vi "FTW-CodeGen-GetTerminals.vi"(0 "PrototypeVI":refnum<vi>, 11 "error in":errorcluster) -> (4 "Terms":T1(array[cluster]), 15 "error out":errorcluster)   [LabVIEW 2014]
panel:
  # "Inputs"
  # "Outputs"
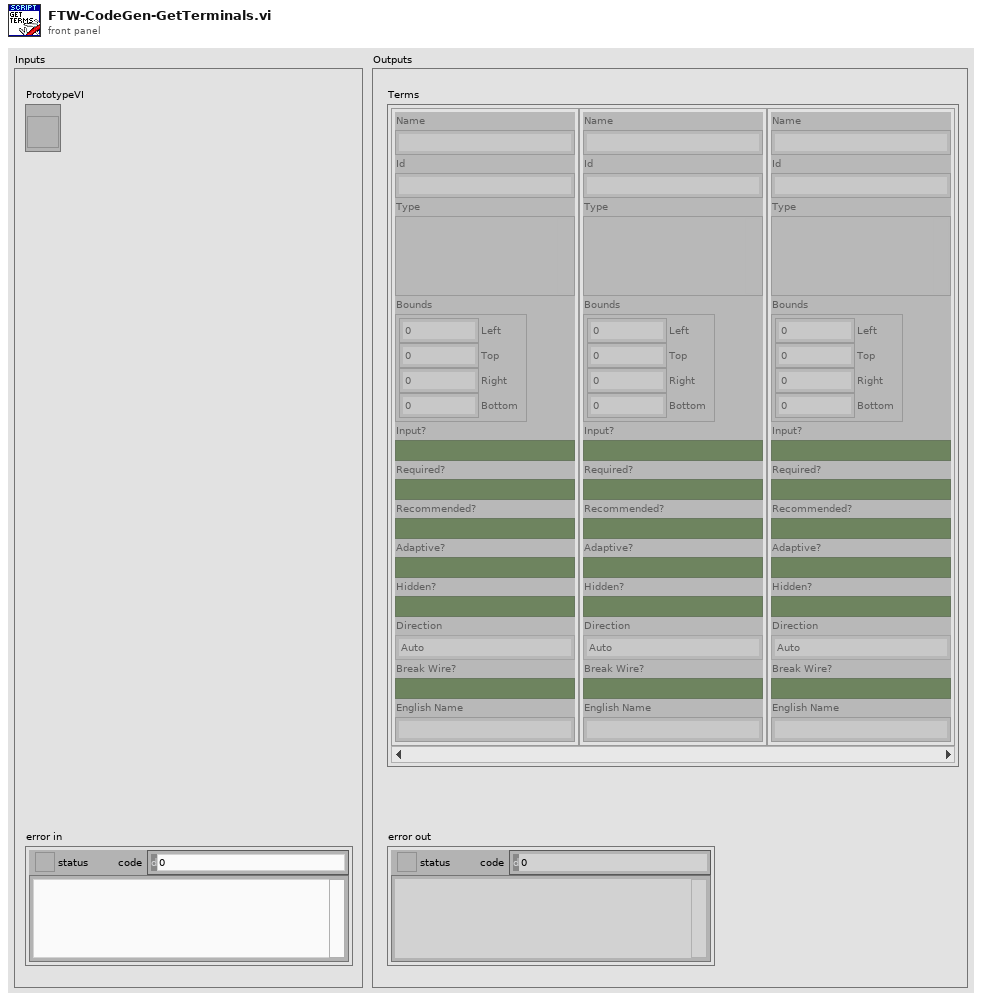
[diagram p1: front panel]
types:
  T1 = cluster{"Name":string, "Id":string, "Type":variant, "Bounds":cluster{"Left":i32, "Top":i32, "Right":i32, "Bottom":i32}, "Input?":bool, "Required?":bool, "Recommended?":bool, "Adaptive?":bool, "Hidden?":bool, "Direction":enum32{"Auto", "Up", "Down", "Left", "Right", "Center"}, "Break Wire?":bool, "English Name":string}[]
  T2 = cluster{"Name":string, "Id":string, "Type":variant, "Bounds":cluster{"Left":i32, "Top":i32, "Right":i32, "Bottom":i32}, "Input?":bool, "Required?":bool, "Recommended?":bool, "Adaptive?":bool, "Hidden?":bool, "Direction":enum32{"Auto", "Up", "Down", "Left", "Right", "Center"}, "Break Wire?":bool, "English Name":string}
  T3 = typedef "LVRectTypeDef.ctl" = cluster{"Left":i16, "Top":i16, "Right":i16, "Bottom":i16}
  T4 = enum16{"Invalid Wire Rule", "Required", "Recommended", "Optional", "Dynamic Dispatch"}[]
  T5 = cluster{"Left":i32, "Top":i32, "Right":i32, "Bottom":i32}[]
  T6 = enum16{"Invalid Wire Rule", "Required", "Recommended", "Optional", "Dynamic Dispatch"}
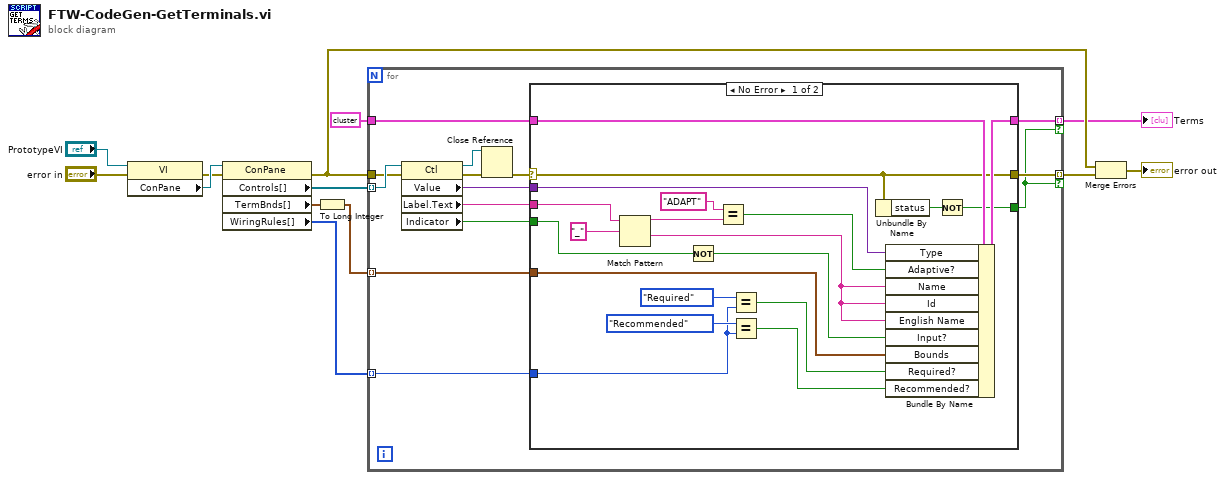
[diagram p0: block diagram]
diagram:
  n1 = property class="VI"(reference="PrototypeVI", error in="error in") -> (error out=w7:errorcluster, "ConPane"=w13:refnum<vi>)  [unwired: 1 out]
  n2 = property class="ConPane"(reference=w13, error in=w7) -> (error out=w6:errorcluster, "Controls[]"=w12:refnum<vi>[], "TermBnds[]"=w9:T3[], "WiringRules[]"=w10:T4)  [unwired: 1 out]
  n3 = To Long Integer(number=w9) -> (32bit integer=w5:T5)
  n4 = for {
    tunnel: w5 -> [w25] mode=indexing
    tunnel: w12 -> [w23] mode=indexing
    tunnel: w10 -> [w24] mode=indexing
    tunnel: T2 {"Name"="", "Id"="", "Type"=variant, "Bounds"={"Left"=0, "Top"=0, "Right"=0, "Bottom"=0}, "Input?"=FALSE, "Required?"=FALSE, "Recommended?"=FALSE, "Adaptive?"=FALSE, "Hidden?"=FALSE, "Direction"=enum."Auto", "Break Wire?"=FALSE, "English Name"=""} ("Term 4") -> [w27]
    tunnel: [w26] -> w4 mode=indexing if=w14
    tunnel: w6 -> [w19]
    tunnel: [w15] -> w8 mode=indexing if=w14
    n5 = property class="Ctl"(reference=w23, error in=w19) -> (reference out=w18:refnum<vi>, error out=w17:errorcluster, "Value"=w22:variant, "Label.Text"=w21:string, "Indicator"=w20:bool)
    n6 = Close Reference(reference=w18, error in (no error)=w17) -> (error out=w16:errorcluster)
    n7 = case shown="No Error" w16 {
      selector: w16 -> [w37 w48]
      tunnel: w27 -> [w47 w49]
      tunnel: [w46 w49] -> w26
      tunnel: w25 -> [w40 _]
      tunnel: w24 -> [w30 _]
      tunnel: w22 -> [w45 _]
      tunnel: w21 -> [w43 _]
      tunnel: w20 -> [w44 _]
      tunnel: [w36 _] -> w14
      tunnel: [w37 w48] -> w15
      frame No Error {
        n8 = Match Pattern(string=w43, regular expression="_") -> (before substring=w35:string, after substring=w41:string)  [unwired: 1 in, 2 out]
        n9 = Not(x=w44) -> (.not. x?=w39:bool)
        n10 = Equal?(x="ADAPT", y=w35) -> (x = y?=w33:bool)
        n11 = Equal?(x=T6."Required" ("Wire Rule"), y=w30) -> (x = y?=w29:bool)
        n12 = Equal?(x=T6."Recommended" ("Wire Rule"), y=w30) -> (x = y?=w28:bool)
        n13 = Unbundle By Name(w37) -> ("status"=w38:bool)
        n14 = Bundle By Name(cluster=w47, "Type"=w45, "Adaptive?"=w33, "Name"=w41, "Id"=w41, "English Name"=w41, "Input?"=w39, "Bounds"=w40, "Required?"=w29, "Recommended?"=w28) -> (w46:T2)
        n15 = Not(x=w38) -> (.not. x?=w36:bool)
      }
      frame Error {
      }
    }
  }
  "Terms" <- w4
  n16 = Merge Errors(w6, w8) -> (→"error out":errorcluster)
